vi "1.Counter.vi"() -> ()   [LabVIEW 2021]
panel:
  out "Boolean":bool
  in  "stop":bool
  out "Counter":dbl
  in  "Limit":dbl
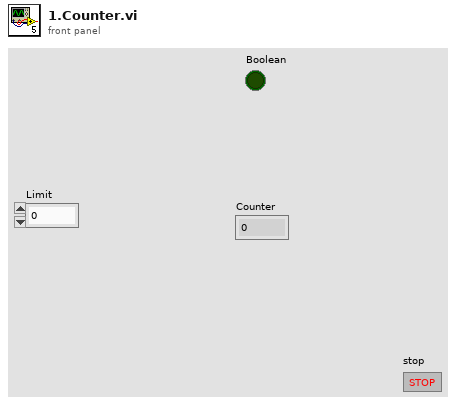
[diagram p1: front panel]
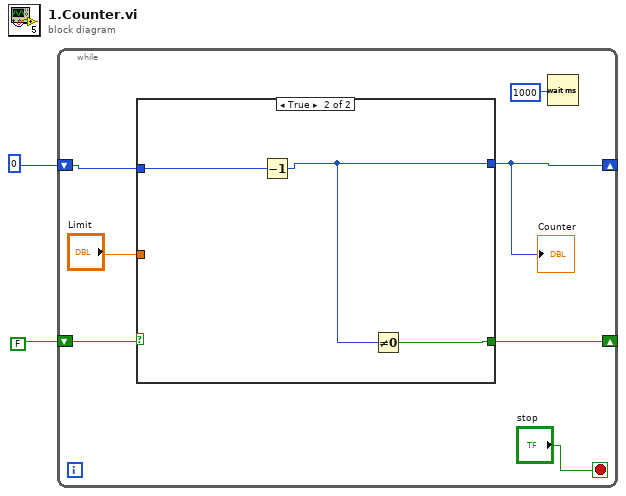
[diagram p0: block diagram]
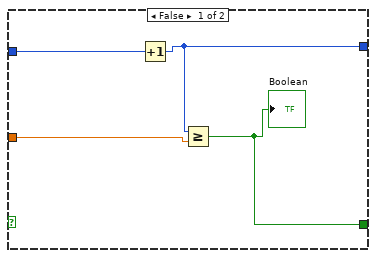
[diagram p2: hidden frame]
diagram:
  n1 = while {
    shift-right: [w7] -> _
    shift-left: 0 -> [w9]
    shift-right: [w8] -> _
    shift-left: FALSE -> [w5]
    stop <- "stop" stop-if-true
    n2 = case shown="True" w5 {
      tunnel: w9 -> [w13 w16]
      tunnel: [w12 w15] -> w7
      tunnel: [w10 w14] -> w8
      tunnel: "Limit" -> [w11 _]
      frame False {
        n3 = Increment(x=w13) -> (x+1=w12:i32)
        n4 = Greater Or Equal?(x=w12, y=w11) -> (x >= y?=w10:bool)
        "Boolean" <- w10
      }
      frame True {
        n5 = Decrement(x=w16) -> (x-1=w15:i32)
        n6 = Not Equal To 0?(x=w15) -> (x != 0?=w14:bool)
      }
    }
    "Counter" <- w7
    n7 = Wait (ms)(milliseconds to wait=1000) -> ()  [unwired: 1 out]
  }
